vi "LowGoalWrapper.vi"(7 "State":T1, 8 "error in":errorcluster) -> (0 "error out":errorcluster)   [LabVIEW 2015]
doc: "Two States: Shoot and Stop\nShoot:\nClapper - Middle\nRoller Motor - Reverse\nRoller Pneumatic - Out\nStop:\nRoller Pneumatic - Middle\nClapper - In\nRoller Motor - Off"
uses:
  LowGoalState.ctl
  DoubleSolenoidAction.ctl
  RollerAction.ctl
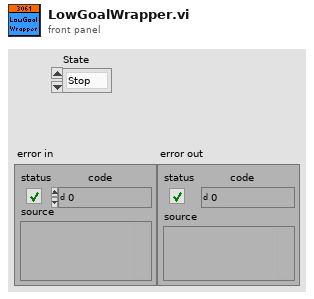
[diagram p1: front panel]
types:
  T1 = typedef "LowGoalState.ctl" = enum16{"Stop", "Shoot"}
  T2 = typedef "RollerAction.ctl" = enum16{"Init", "Off", "Forward", "Reverse"}
  T3 = typedef "DoubleSolenoidAction.ctl" = enum16{"Init", "Middle", "In", "Out"}
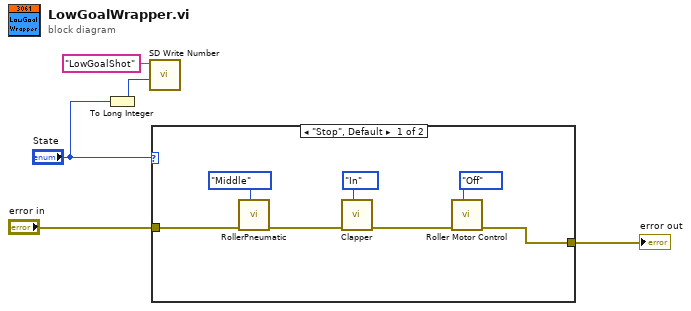
[diagram p0: block diagram]
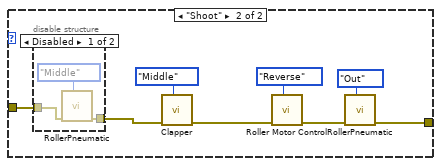
[diagram p2: hidden frame]
diagram:
  n1 = To Long Integer(number="State") -> (32bit integer=w3:i32)
  n2 = call <vilib>:"SD Write Number.vi"("Numeric"=w3, "Name"="LowGoalShot") -> ()  [unwired: 8 in, 2 out]
  n3 = case shown="\"Stop\", Default" "State" {
    tunnel: "error in" -> [w7 w14]
    tunnel: [w6 w13] -> w4
    frame "Stop", Default {
      n4 = call "RollerPneumatic.vi"("State"=DoubleSolenoidAction."Middle", "Error in"=w7) -> ("Error out"=w8:errorcluster)  [unwired: 9 in]
      n5 = call "Clapper.vi"("State"=DoubleSolenoidAction."In", "Error in"=w8) -> ("Error out"=w9:errorcluster)  [unwired: 9 in]
      n6 = call "Roller Motor Control.vi"("Action"=RollerAction."Off", "Error in"=w9) -> ("Error out"=w6:errorcluster)  [unwired: 9 in]
    }
    frame "Shoot" {
      n7 = disable-structure shown="Disabled" {
        disable-tunnel: [w22 _] -> w15
        disable-tunnel: w14 -> [w21 _]
        frame Disabled {
          n8 = call "RollerPneumatic.vi"("State"=DoubleSolenoidAction."Middle", "Error in"=w21) -> ("Error out"=w22:errorcluster)  [unwired: 9 in]
        }
        frame Enabled {
        }
      }
      n9 = call "Clapper.vi"("State"=DoubleSolenoidAction."Middle", "Error in"=w15) -> ("Error out"=w18:errorcluster)  [unwired: 9 in]
      n10 = call "Roller Motor Control.vi"("Action"=RollerAction."Reverse", "Error in"=w18) -> ("Error out"=w17:errorcluster)  [unwired: 9 in]
      n11 = call "RollerPneumatic.vi"("State"=DoubleSolenoidAction."Out", "Error in"=w17) -> ("Error out"=w13:errorcluster)  [unwired: 9 in]
    }
  }
  "error out" <- w4
